vi "Untitled 2.vi"() -> ()   [LabVIEW 2019]
uses:
  Control 1.ctl
panel:
  in  "String":string
  out "Boolean":bool
  in  "zadanie 2":bool
  out "date/time string":string
  in  "zadanie 1":bool
  in  "stop":bool
  out "x+1":i32
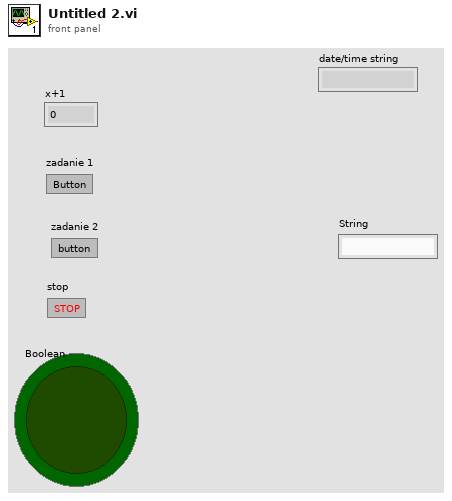
[diagram p1: front panel]
types:
  T1 = typedef "Control 1.ctl" = enum16{"init", "idle", "zadanie 1", "stop"}
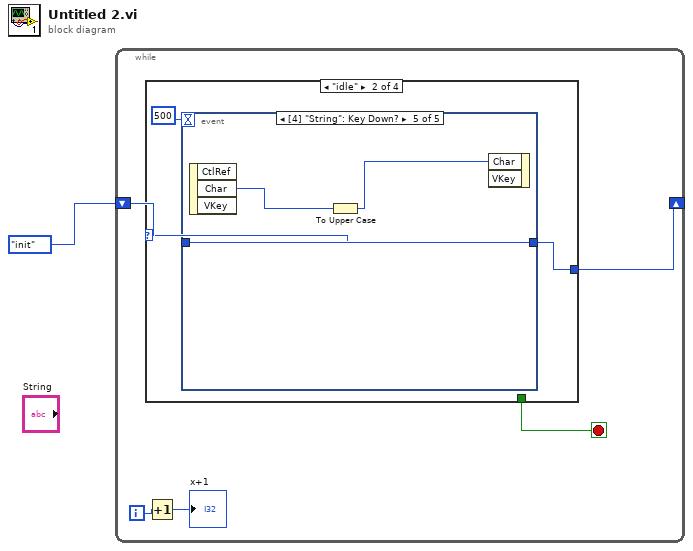
[diagram p0: block diagram]
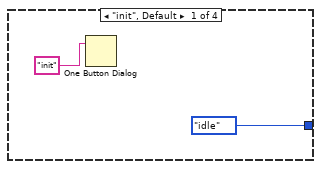
[diagram p2: hidden frame]
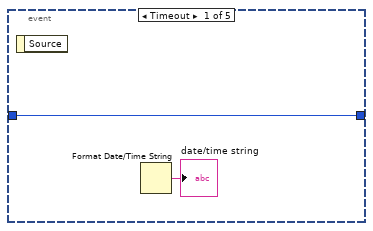
[diagram p3: hidden frame]
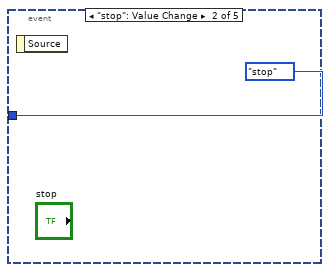
[diagram p4: hidden frame]
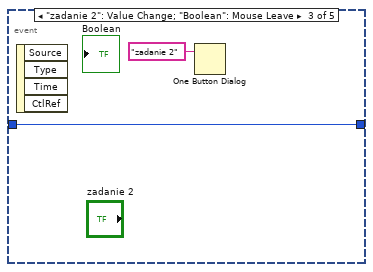
[diagram p5: hidden frame]
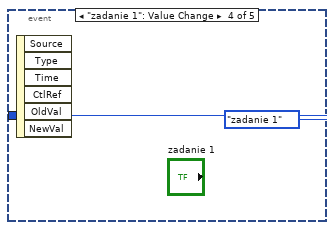
[diagram p6: hidden frame]
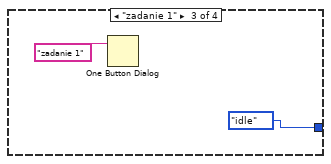
[diagram p7: hidden frame]
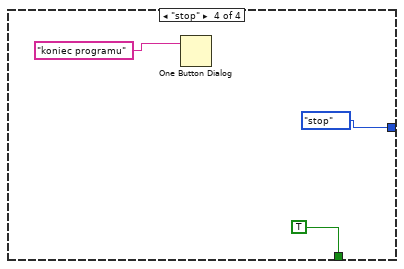
[diagram p8: hidden frame]
diagram:
  n1 = while {
    shift-right: [w5] -> _
    shift-left: Control_1."init" -> [w6]
    i -> [w4]
    stop <- w2 stop-if-true
    n2 = case shown="\"idle\"" w6 {
      selector: w6 -> [_ w10 _ _]
      tunnel: [Control_1."idle" w11 Control_1."idle" Control_1."stop"] -> w5
      tunnel: [_ _ _ TRUE] -> w2
      frame "init", Default {
        n3 = One Button Dialog(message="init") -> ()  [unwired: 1 in, 1 out]
      }
      frame "idle" {
        n4 = event shown="[4] \"String\": Key Down?" {
          selector: _ -> [_ _ _ _ _]
          dyn-events: _ -> [_ _ _ _ _]
          timeout: 500 -> [_ _ _ _ _]
          tunnel: [w13 Control_1."stop" w16 Control_1."zadanie 1" w18] -> w11
          tunnel: w10 -> [w13 _ w16 _ w18]
          event Timeout {
            n5 = event-data() -> ()  [unwired: 1 in, 1 out]
            n6 = Format Date/Time String() -> (date/time string=→"date/time string":string)  [unwired: 3 in]
          }
          event "stop": Value Change {
            n7 = event-data() -> ()  [unwired: 1 in, 1 out]
          }
          event "zadanie 2": Value Change; "Boolean": Mouse Leave {
            n8 = event-data() -> ()  [unwired: 1 in, 4 out]
            n9 = One Button Dialog(message="zadanie 2") -> ()  [unwired: 1 in, 1 out]
          }
          event "zadanie 1": Value Change {
            n10 = event-data() -> ()  [unwired: 1 in, 6 out]
          }
          event "String": Key Down? {
            n11 = event-data() -> ("Char"=w20:i16)  [unwired: 1 in, 2 out]
            n12 = To Upper Case(1:w20) -> (0:w19:i16)
            n13 = event-data("Char"=w19) -> ()  [unwired: 2 in, 1 out]
          }
        }
      }
      frame "zadanie 1" {
        n14 = One Button Dialog(message="zadanie 1") -> ()  [unwired: 1 in, 1 out]
      }
      frame "stop" {
        n15 = One Button Dialog(message="koniec programu") -> ()  [unwired: 1 in, 1 out]
      }
    }
    n16 = Increment(x=w4) -> (x+1=→"x+1":i32)
  }
